vi "CS-4 Get Stb.vi"(4 "error in (no error)":errorcluster, 7 "VISA session":refnum<visa-resource-name>) -> (0 "error out":errorcluster, 1 "Off Line":bool, 2 "stb":i32, 3 "dup VISA session":refnum<visa-resource-name>)   [LabVIEW 2016]
doc: "CS-4 Get Stb.vi will return the status byte and the off line flag. If Local or Menu has been selected on the instrument keypad the 'off line' flag will be TRUE."
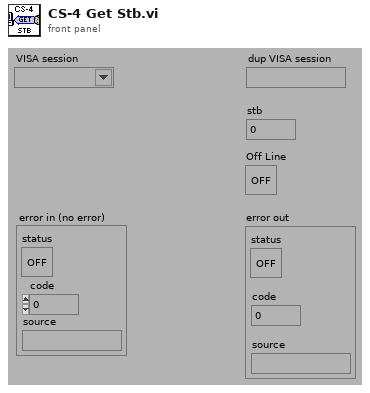
[diagram p1: front panel]
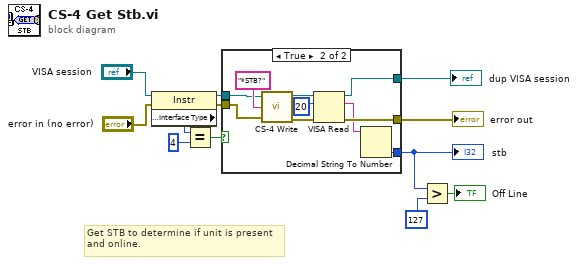
[diagram p0: block diagram]
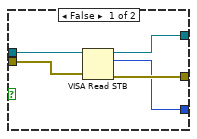
[diagram p2: hidden frame]
diagram:
  # "Get STB to determine if unit is present\nand online."
  n1 = property class="Instr"(reference="VISA session", error in="error in (no error)") -> (reference out=w8:refnum<visa-resource-name>, error out=w7:errorcluster, "Interface Information:Interface Type"=w11:u16)
  n2 = Equal?(x=w11, y=u16 4) -> (x = y?=w9:bool)
  n3 = case shown="True" w9 {
    tunnel: [w15 w27] -> w6
    tunnel: [w14 w25] -> w3
    tunnel: w8 -> [w17 w20]
    tunnel: w7 -> [w16 w19]
    tunnel: [w13 w18] -> w4
    frame False {
      n4 = VISA Read STB(8:w16, 11:w17) -> (0:w15:errorcluster, 2:w14:u16, 3:w13:refnum<visa-resource-name>)
    }
    frame True {
      n5 = call "CS-4 Write.vi"("error in (no error)"=w19, "write buffer (\"\")"="*STB?" ("write buffer (\"\")"), "VISA session"=w20) -> ("error out"=w23:errorcluster, "dup VISA session"=w22:refnum<visa-resource-name>)  [unwired: 1 out]
      n6 = VISA Read(VISA resource name=w22, byte count=u32 20 ("byte count (0)"), error in (no error)=w23) -> (VISA resource name out=w18:refnum<visa-resource-name>, read buffer=w24:string, error out=w27:errorcluster)  [unwired: 1 out]
      n7 = Decimal String To Number(string=w24) -> (number=w25:i32)  [unwired: 2 in, 1 out]
    }
  }
  "stb" <- w3
  "error out" <- w6
  "dup VISA session" <- w4
  n8 = Greater?(x=w3, y=127) -> (0:→"Off Line":bool)
